vi "Set Ramp Rate.vi"(8 "error in":errorcluster, 11 "6700C in":refnum<class "6700C.lvclass">) -> (0 "error out":errorcluster, 3 "6700C out":refnum<class "6700C.lvclass">)   [LabVIEW 2019, in "6700C.lvlib" / "6700C.lvclass"]
uses:
  Library/6700C.lvclass
  C:/Users/Public/Documents/Development/builds/Instruments/PowerSupply.lvlibp/Library/PowerSupply.lvclass
  Library/6700C.lvclass/6700C.ctl
  Accessors/Read Local Resource.vi
  Accessors/Write Local Resource.vi
  builds/Instruments/PowerSupply.lvlibp/Accessors/Read Active Channel.vi
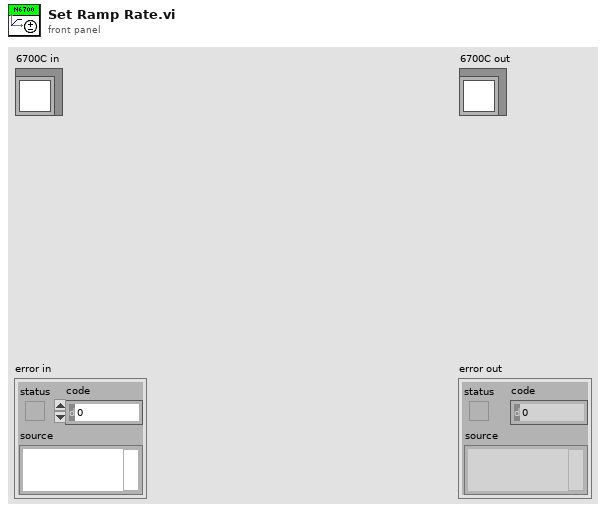
[diagram p1: front panel]
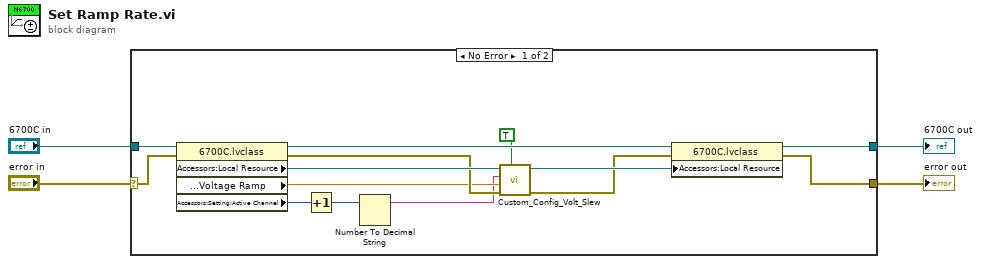
[diagram p0: block diagram]
diagram:
  n1 = case shown="No Error" "error in" {
    selector: "error in" -> [w15 w20]
    tunnel: [w16 w20] -> w3
    tunnel: [w17 w19] -> w1
    tunnel: "6700C in" -> [w18 w19]
    frame No Error {
      n2 = property class="6700C.lvclass"(reference=w18, error in=w15) -> (reference out=w12:refnum<class "6700C.lvclass">, error out=w13:errorcluster, "Accessors:Local Resource"=w14:refnum<visa-resource-name>, "Accessors:Setting:Ramp:Voltage Ramp"=w9:dbl, "Accessors:Setting:Active Channel"=w8:u32)
      n3 = Increment(x=w8) -> (x+1=w6:u32)
      n4 = Number To Decimal String(number=w6) -> (decimal integer string=w7:string)  [unwired: 1 in]
      n5 = call "Custom_Config_Volt_Slew.vi"("Enable Voltage Slew Rate Override (False)"=TRUE, "error in (no error)"=w13, "Voltage Slew Rate (9.9E+37 A/s)"=w9, "Channel Name (1)"=w7, "VISA resource name"=w14) -> ("error out"=w10:errorcluster, "VISA resource name out"=w11:refnum<visa-resource-name>)  [unwired: 5 in]
      n6 = property class="6700C.lvclass"(reference=w12, error in=w10, "Accessors:Local Resource"=w11) -> (reference out=w17:refnum<class "6700C.lvclass">, error out=w16:errorcluster)
    }
    frame Error {
    }
  }
  "error out" <- w3
  "6700C out" <- w1
